vi "PS Control.vi"() -> ()   [LabVIEW 2025]
doc: "Author: Scott Hannahs <sth@magnet.fsu.edu>\n\nThis software is licensed for use under the “MIT License\"\nCopyright (c) 2025 Scott Hannahs, sth@sth@magnet.sthnet.net\n\nPermission is hereby granted, free of charge, to any person obtaining a copy of this software and associated documentation files (the \"Software\"), to deal in the Software without restriction, including without limitation the rights to use, copy, modify, merge, publish, distribute, sublicense, and/or sell copies of the Software, and to permit persons to whom the Software is furnished to do so, subject to the following conditions: The above copyright notice and this permission notice shall be included in all copies or substantial portions of the Software.\n\nTHE SOFTWARE IS PROVIDED \"AS IS\", WITHOUT WARRANTY OF ANY KIND, EXPRESS OR IMPLIED, INCLUDING BUT NOT LIMITED TO THE WARRANTIES OF MERCHANTABILITY, FITNESS FOR A PARTICULAR PURPOSE AND NONINFRINGEMENT. IN NO EVENT SHALL THE AUTHORS OR COPYRIGHT HOLDERS BE LIABLE FOR ANY CLAIM, DAMAGES OR OTHER LIABILITY, WHETHER IN AN ACTION OF CONTRACT, TORT OR OTHERWISE, ARISING FROM, OUT OF OR IN CONNECTION WITH THE SOFTWARE OR THE USE OR OTHER DEALINGS IN THE SOFTWARE."
uses:
  Sub Controls/PS Status.ctl
  PS Comm Globals.vi
panel:
  out "Status":T1
  in  "Slew Rate [T/min]":dbl=1.0 caption="(7.055) Max)" min=0.001 max=50.0 step=0.01 format="%.3f"
  in  "Slew Rate [A/s]":dbl=200.0 caption="(200.0) Max)" min=0.1 max=4000.0 step=10.0 format="%.1f"
  out "Read Loop Ref":refnum<vi>
  out "SC Current [kA]":dbl format="%.5f"
  in  "dup VI reference":refnum<vi>
  in  "Setpoint [kA]":dbl caption="(59.0) Max)" min=-59.0 max=59.0 format="%.5f"
  in  "Setpoint [T]":dbl caption="(34.68) Max)" min=-34.679602421022246 max=34.679602421022246 format="%.5f"
  in  "Pause":bool
  out "Current [kA]":dbl format="%.5f"
  out "Field [T]":dbl caption="Current [kA]" format="%.5f"
  in  "Units":enum32{"tesla", "kAmps"}(radio) caption="tesla            kAmps"
  in  "stop":bool
  in  "Ramp":bool
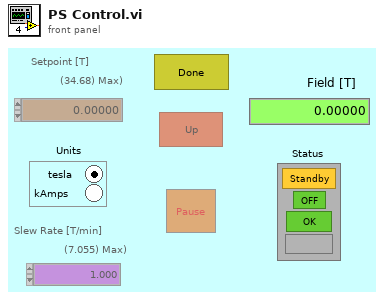
[diagram p1: front panel]
types:
  T1 = typedef "PS Status.ctl" = cluster{"PS On":bool, "PS Fault":bool, "Ramp Status":u16, "Cell Control":bool}
  T2 = cluster{"Control Name":string, "Type Descriptor":i16[], "Flattened Data":string}
  T3 = cluster{"Minimum":dbl, "Maximum":dbl, "Increment":dbl}
  T4 = cluster{string, "type string":i16[], "data string":string}
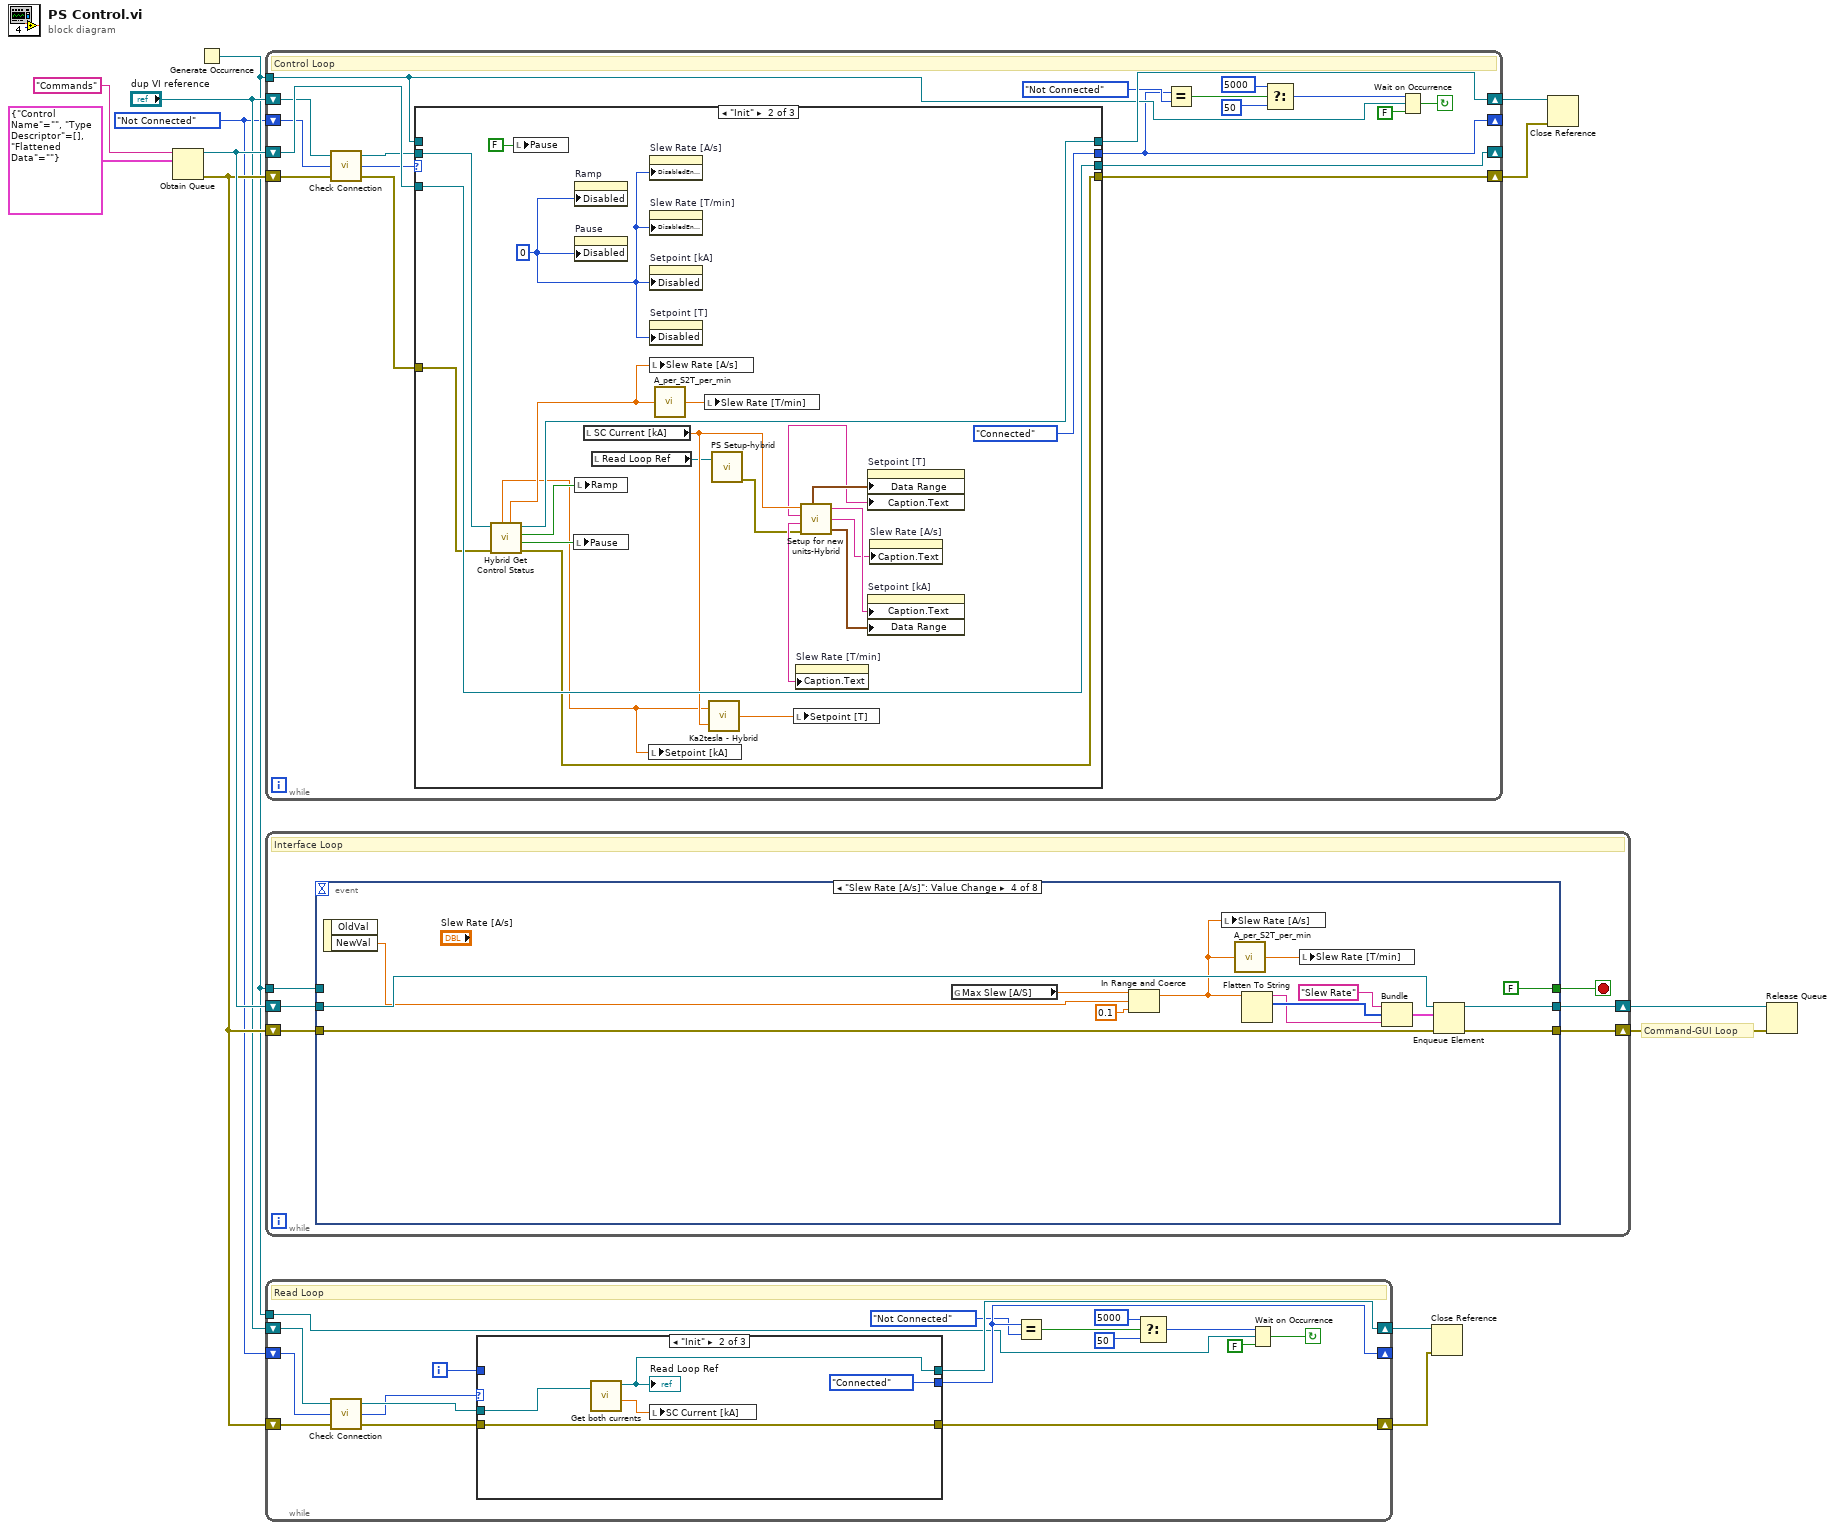
[diagram p0: block diagram]
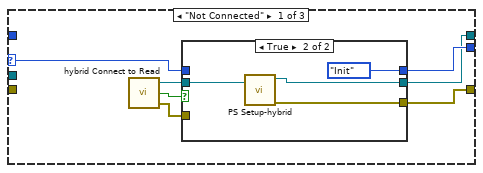
[diagram p2: hidden frame]
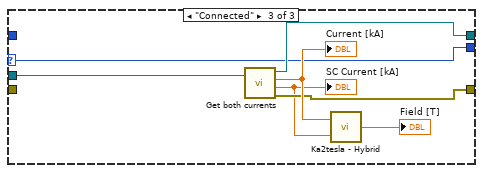
[diagram p4: hidden frame]
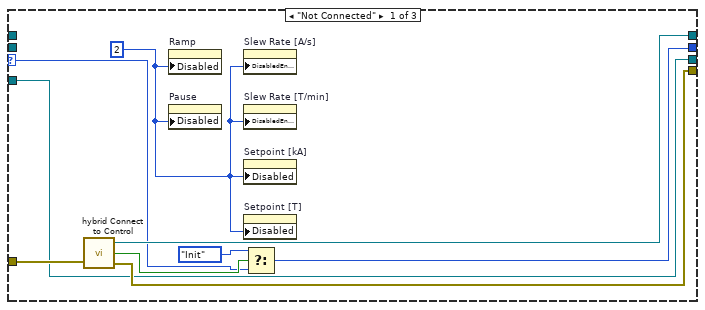
[diagram p5: hidden frame]
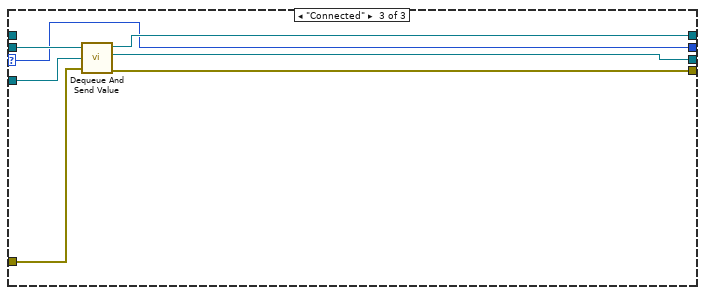
[diagram p6: hidden frame]
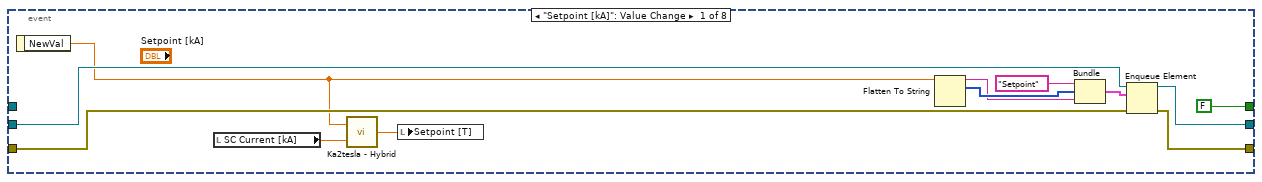
[diagram p7: hidden frame]
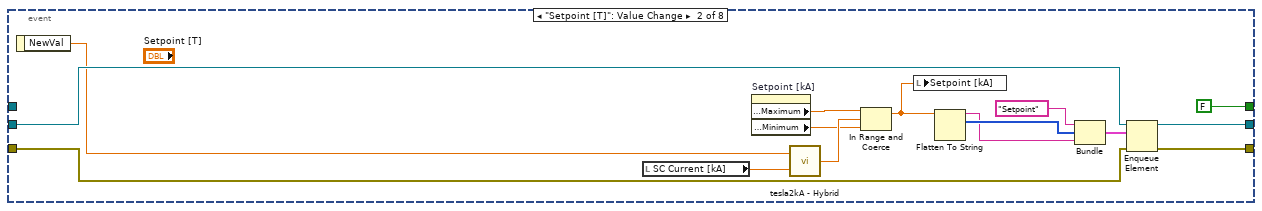
[diagram p8: hidden frame]
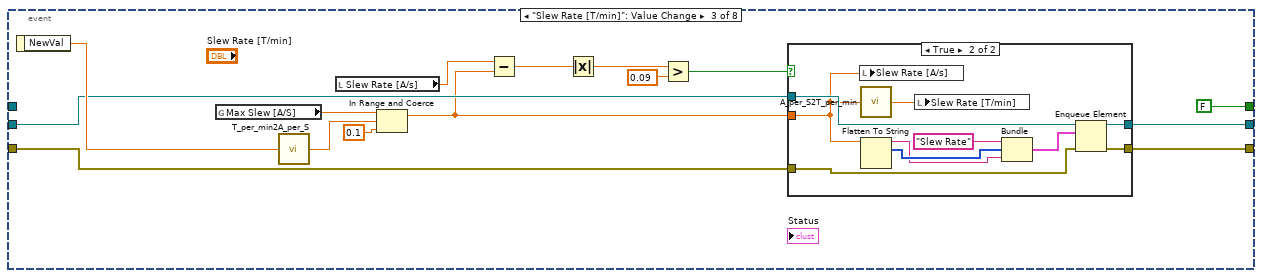
[diagram p9: hidden frame]
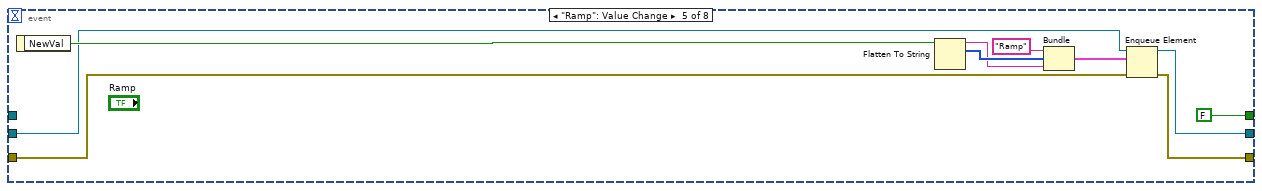
[diagram p11: hidden frame]
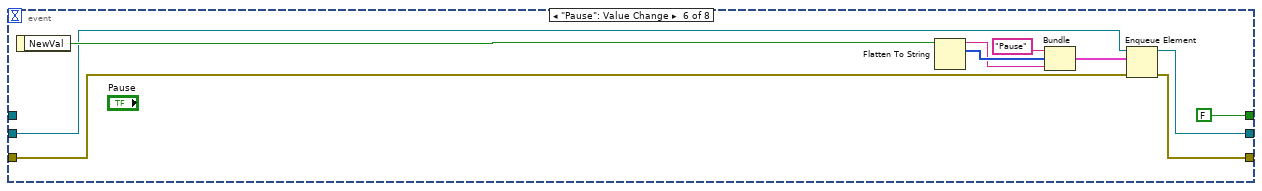
[diagram p12: hidden frame]
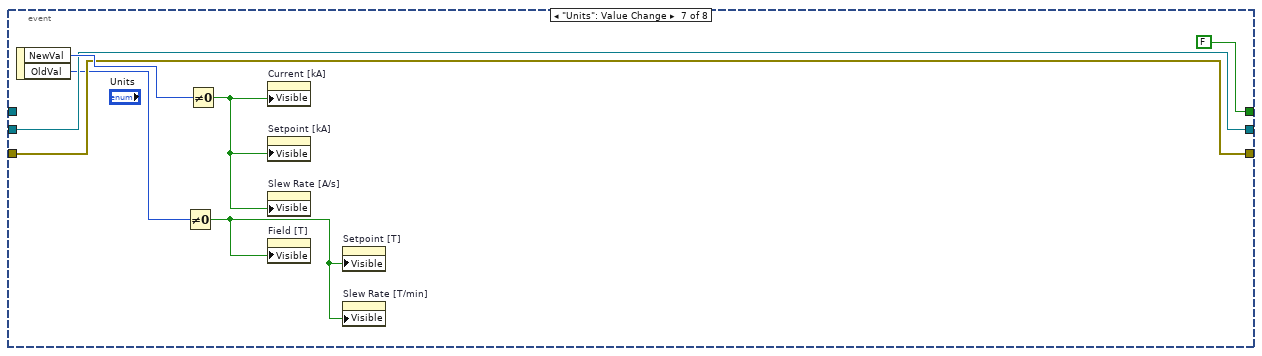
[diagram p13: hidden frame]
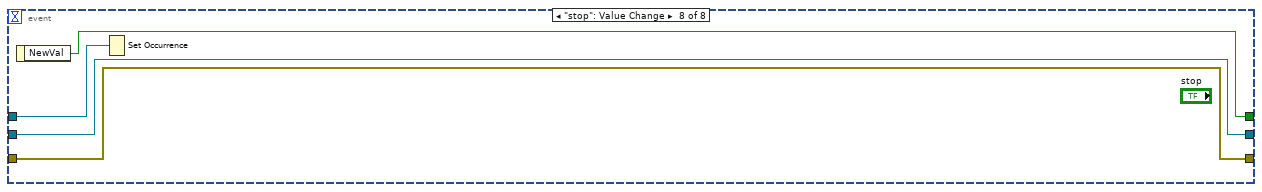
[diagram p14: hidden frame]
diagram:
  w1 = enum16{"Not Connected", "Init", "Connected"}."Not Connected"
  # "Command-GUI Loop"
  n1 = Obtain Queue(name (unnamed)="Commands", element data type=T2 {"Control Name"="", "Type Descriptor"=[], "Flattened Data"=""}) -> (queue out=w11:refnum<queue>, error out=w6:errorcluster)  [unwired: 3 in, 1 out]
  n2 = Generate Occurrence() -> (w2:refnum<k4>)
  n3 = while {
    shift-right: [w32] -> w8
    shift-left: "dup VI reference" -> [w27]
    shift-right: [w31] -> w7
    shift-left: w6 -> [w26]
    shift-right: [w29] -> _
    shift-left: w11 -> [w30]
    tunnel: w2 -> [w22]
    shift-right: [w15] -> _
    shift-left: w1 -> [w24]
    stop <- w21 continue-if-true
    # "Control Loop"
    n4 = call "Check Connection.vi"("error In"=w26, "State In"=w24, "VI reference"=w27) -> ("error out"=w25:errorcluster, "State Out"=w23:enum16{"Not Connected", "Init", "Connected"}, "dup VI reference"=w28:refnum<vi>)
    n5 = case shown="\"Init\"" w23 {
      selector: w23 -> [w35 _ w65]
      tunnel: [w41 w54 w66] -> w32
      tunnel: w25 -> [w40 w53 w69]
      tunnel: [w39 w52 w67] -> w31
      tunnel: w30 -> [w38 w63 w71]
      tunnel: [w38 w63 w70] -> w29
      tunnel: w28 -> [_ w64 w68]
      tunnel: w22 -> [_ _ _]
      tunnel: [w34 enum16{"Not Connected", "Init", "Connected"}."Connected" ("f") w65] -> w15
      frame "Not Connected" {
        w33 = u8 2 ("Disabled")
        n6 = call "hybrid Connect to Control.vi"("error in"=w40) -> ("VI Refnum"=w41:refnum<vi>, "Success"=w37:bool, "error out"=w39:errorcluster)  [unwired: 1 in]
        n7 = property on="Ramp" class="Bool (strict)"("Disabled"=w33) -> ()  [unwired: 2 in, 2 out]
        n8 = property on="Pause" class="Bool (strict)"("Disabled"=w33) -> ()  [unwired: 2 in, 2 out]
        n9 = property on="Slew Rate [A/s]" class="DigNum (strict)"("DisabledEnum"=w33) -> ()  [unwired: 2 in, 2 out]
        n10 = property on="Slew Rate [T/min]" class="DigNum (strict)"("DisabledEnum"=w33) -> ()  [unwired: 2 in, 2 out]
        n11 = property on="Setpoint [kA]" class="DigNum (strict)"("Disabled"=w33) -> ()  [unwired: 2 in, 2 out]
        n12 = property on="Setpoint [T]" class="DigNum (strict)"("Disabled"=w33) -> ()  [unwired: 2 in, 2 out]
        n13 = Select(t=enum16{"Not Connected", "Init", "Connected"}."Init", s=w37, f=w35) -> (s? t:f=w34:enum16{"Not Connected", "Init", "Connected"})
      }
      frame "Init" {
        w49 = u8 0 ("Disabled")
        n14 = call "Hybrid Get Control Status.vi"("error in (no error)"=w53, "VI in"=w64) -> ("error out"=w52:errorcluster, "Pause"=w50:bool, "Ramp"=w51:bool, "VI out"=w54:refnum<vi>, "Slew Rate [A/s]"=w45:dbl, "Setpoint"=w44:dbl)  [unwired: 4 in]
        n15 = local write "Pause"(FALSE ("Pause")) -> ()
        n16 = local write "Pause"(w50) -> ()
        n17 = property on="Ramp" class="Bool (strict)"("Disabled"=w49) -> ()  [unwired: 2 in, 2 out]
        n18 = property on="Pause" class="Bool (strict)"("Disabled"=w49) -> ()  [unwired: 2 in, 2 out]
        n19 = local write "Ramp"(w51) -> ()
        n20 = local read "SC Current [kA]"() -> (w61:dbl)
        n21 = local read "Read Loop Ref"() -> (w43:refnum<vi>)
        n22 = local write "Setpoint [kA]"(w44) -> ()
        n23 = property on="Slew Rate [A/s]" class="DigNum (strict)"("DisabledEnum"=w49) -> ()  [unwired: 2 in, 2 out]
        n24 = property on="Slew Rate [T/min]" class="DigNum (strict)"("DisabledEnum"=w49) -> ()  [unwired: 2 in, 2 out]
        n25 = property on="Setpoint [kA]" class="DigNum (strict)"("Disabled"=w49) -> ()  [unwired: 2 in, 2 out]
        n26 = property on="Setpoint [T]" class="DigNum (strict)"("Disabled"=w49) -> ()  [unwired: 2 in, 2 out]
        n27 = local write "Slew Rate [A/s]"(w45) -> ()
        n28 = call "A_per_S2T_per_min.vi"("A/sec"=w45) -> ("T/min"=w46:dbl)
        n29 = local write "Slew Rate [T/min]"(w46) -> ()
        n30 = call "Ka2tesla - Hybrid.vi"("SC Current [kA]"=w61, "Current [KA]"=w44) -> ("Field"=w56:dbl)
        n31 = call "PS Setup-hybrid.vi"("vi reference"=w43) -> ("error out"=w42:errorcluster)  [unwired: 4 in, 2 out]
        n32 = local write "Setpoint [T]"(w56) -> ()
        n33 = call "Setup for new units-Hybrid.vi"("SC Current [kA]"=w61, "error in (no error)"=w42) -> ("Field Setpoint Caption"=w57:string, "Field Slew Rate Caption"=w47:string, "Field Range"=w58:T3, "Current Setpoint Caption"=w60:string, "Current Slew Rate Caption"=w48:string, "Current Range"=w59:T3)
        n34 = property on="Slew Rate [T/min]" class="DigNum (strict)"("Caption.Text"=w47) -> ()  [unwired: 2 in, 2 out]
        n35 = property on="Setpoint [T]" class="DigNum (strict)"("Data Range"=w58, "Caption.Text"=w57) -> ()  [unwired: 2 in, 2 out]
        n36 = property on="Setpoint [kA]" class="DigNum (strict)"("Caption.Text"=w60, "Data Range"=w59) -> ()  [unwired: 2 in, 2 out]
        n37 = property on="Slew Rate [A/s]" class="DigNum (strict)"("Caption.Text"=w48) -> ()  [unwired: 2 in, 2 out]
      }
      frame "Connected" {
        n38 = call "Dequeue And Send Value.vi"("VI reference"=w68, "queue in"=w71, "error in"=w69) -> ("dup VI Refnum"=w66:refnum<vi>, "queue out"=w70:refnum<queue>, "error out"=w67:errorcluster)  [unwired: 1 out]
      }
    }
    n39 = Equal?(x=w15, y=enum16{"Not Connected", "Init", "Connected"}."Not Connected") -> (x = y?=w16:bool)
    n40 = Select(t=5000 ("ms timeout (-1)"), s=w16, f=50 ("ms timeout (-1)")) -> (s? t:f=w14:i32)
    n41 = Wait on Occurrence(1:FALSE ("ignore previous (T)"), 2:w22, 3:w14) -> (0:w21:bool)
  }
  n42 = while {
    tunnel: w2 -> [w76]
    shift-right: [w74] -> w9
    shift-left: w11 -> [w75]
    shift-right: [w72] -> w10
    shift-left: w6 -> [w73]
    stop <- w77 stop-if-true
    # "Interface Loop"
    n43 = event shown="[3] \"Slew Rate [A/s]\": Value Change" {
      selector: _ -> [_ _ _ _ _ _ _ _]
      dyn-events: _ -> [_ _ _ _ _ _ _ _]
      timeout: _ -> [_ _ _ _ _ _ _ _]
      tunnel: [FALSE ("NewVal") FALSE ("NewVal") FALSE ("NewVal") FALSE ("NewVal") FALSE ("NewVal") FALSE ("NewVal") FALSE ("NewVal") w176] -> w77
      tunnel: w73 -> [w84 w99 w115 w140 w150 w160 w170 w173]
      tunnel: w76 -> [_ _ _ _ _ _ _ w175]
      tunnel: w75 -> [w87 w102 w113 w144 w152 w162 w171 w174]
      tunnel: [w85 w100 w112 w141 w151 w161 w171 w174] -> w74
      tunnel: [w83 w98 w114 w139 w149 w159 w170 w173] -> w72
      event "Setpoint [kA]": Value Change {
        n44 = event-data() -> ("NewVal"=w79:dbl)  [unwired: 1 in]
        n45 = local read "SC Current [kA]"() -> (w78:dbl)
        n46 = call "Ka2tesla - Hybrid.vi"("SC Current [kA]"=w78, "Current [KA]"=w79) -> ("Field"=w80:dbl)
        n47 = local write "Setpoint [T]"(w80) -> ()
        n48 = Flatten To String(anything=w79) -> (data string=w88:string, type string=w89:i16[])  [unwired: 3 in, 1 out]
        n49 = Bundle("Setpoint", "type string"=w89, "data string"=w88) -> (w86:T4)  [unwired: 1 in]
        n50 = Enqueue Element(queue=w87, element=w86, error in (no error)=w84) -> (queue out=w85:refnum<queue>, error out=w83:errorcluster)  [unwired: 1 in, 1 out]
      }
      event "Setpoint [T]": Value Change {
        n51 = event-data() -> ("NewVal"=w95:dbl)  [unwired: 1 in]
        n52 = local read "SC Current [kA]"() -> (w90:dbl)
        n53 = property on="Setpoint [kA]" class="DigNum (strict)"() -> ("Data Range:Maximum"=w92:dbl, "Data Range:Minimum"=w91:dbl)  [unwired: 2 in, 2 out]
        n54 = call "tesla2kA - Hybrid.vi"("SC Current [kA]"=w90, "Magnet Field [T]"=w95) -> ("Current [kA]"=w94:dbl)
        n55 = In Range and Coerce(upper limit=w92, x=w94, lower limit=w91) -> (coerced(x)=w93:dbl)  [unwired: 1 out]
        n56 = local write "Setpoint [kA]"(w93) -> ()
        n57 = Flatten To String(anything=w93) -> (data string=w103:string, type string=w104:i16[])  [unwired: 3 in, 1 out]
        n58 = Bundle("Setpoint", "type string"=w104, "data string"=w103) -> (w101:T4)  [unwired: 1 in]
        n59 = Enqueue Element(queue=w102, element=w101, error in (no error)=w99) -> (queue out=w100:refnum<queue>, error out=w98:errorcluster)  [unwired: 1 in, 1 out]
      }
      event "Slew Rate [T/min]": Value Change {
        n60 = event-data() -> ("NewVal"=w119:dbl)  [unwired: 1 in]
        n61 = global read "PS Comm Globals.vi" "Max Slew [A/S]"() -> (w117:dbl)
        n62 = call "T_per_min2A_per_S.vi"("T/min"=w119) -> ("A/sec"=w116:dbl)
        n63 = local read "Slew Rate [A/s]"() -> (w109:dbl)
        n64 = In Range and Coerce(upper limit=w117, x=w116, lower limit=0.1) -> (coerced(x)=w110:dbl)  [unwired: 1 out]
        n65 = Subtract(x=w109, y=w110) -> (x-y=w108:dbl)
        n66 = Absolute Value(x=w108) -> (abs(x)=w107:dbl)
        n67 = Greater?(x=w107, y=0.09) -> (0:w105:bool)
        n68 = case shown="True" w105 {
          tunnel: w115 -> [w120 w126]
          tunnel: [w120 w125] -> w114
          tunnel: w113 -> [w121 w124]
          tunnel: [w121 w123] -> w112
          tunnel: w110 -> [_ w122]
          frame False {
          }
          frame True {
            n69 = local write "Slew Rate [A/s]"(w122) -> ()
            n70 = call "A_per_S2T_per_min.vi"("A/sec"=w122) -> ("T/min"=w131:dbl)
            n71 = Flatten To String(anything=w122) -> (data string=w129:string, type string=w130:i16[])  [unwired: 3 in, 1 out]
            n72 = local write "Slew Rate [T/min]"(w131) -> ()
            n73 = Bundle("Slew Rate", "type string"=w130, "data string"=w129) -> (w127:T4)  [unwired: 1 in]
            n74 = Enqueue Element(queue=w124, element=w127, error in (no error)=w126) -> (queue out=w123:refnum<queue>, error out=w125:errorcluster)  [unwired: 1 in, 1 out]
          }
        }
      }
      event "Slew Rate [A/s]": Value Change {
        n75 = event-data() -> ("NewVal"=w143:dbl)  [unwired: 1 in, 1 out]
        n76 = global read "PS Comm Globals.vi" "Max Slew [A/S]"() -> (w133:dbl)
        n77 = In Range and Coerce(upper limit=w133, x=w143, lower limit=0.1) -> (coerced(x)=w134:dbl)  [unwired: 1 out]
        n78 = local write "Slew Rate [A/s]"(w134) -> ()
        n79 = call "A_per_S2T_per_min.vi"("A/sec"=w134) -> ("T/min"=w145:dbl)
        n80 = Flatten To String(anything=w134) -> (data string=w137:string, type string=w138:i16[])  [unwired: 3 in, 1 out]
        n81 = local write "Slew Rate [T/min]"(w145) -> ()
        n82 = Bundle("Slew Rate", "type string"=w138, "data string"=w137) -> (w135:T4)  [unwired: 1 in]
        n83 = Enqueue Element(queue=w144, element=w135, error in (no error)=w140) -> (queue out=w141:refnum<queue>, error out=w139:errorcluster)  [unwired: 1 in, 1 out]
      }
      event "Ramp": Value Change {
        n84 = event-data() -> ("NewVal"=w155:bool)  [unwired: 1 in]
        n85 = Flatten To String(anything=w155) -> (data string=w153:string, type string=w154:i16[])  [unwired: 3 in, 1 out]
        n86 = Bundle("Ramp", "type string"=w154, "data string"=w153) -> (w147:T4)  [unwired: 1 in]
        n87 = Enqueue Element(queue=w152, element=w147, error in (no error)=w150) -> (queue out=w151:refnum<queue>, error out=w149:errorcluster)  [unwired: 1 in, 1 out]
      }
      event "Pause": Value Change {
        n88 = event-data() -> ("NewVal"=w165:bool)  [unwired: 1 in]
        n89 = Flatten To String(anything=w165) -> (data string=w163:string, type string=w164:i16[])  [unwired: 3 in, 1 out]
        n90 = Bundle("Pause", "type string"=w164, "data string"=w163) -> (w157:T4)  [unwired: 1 in]
        n91 = Enqueue Element(queue=w162, element=w157, error in (no error)=w160) -> (queue out=w161:refnum<queue>, error out=w159:errorcluster)  [unwired: 1 in, 1 out]
      }
      event "Units": Value Change {
        n92 = event-data() -> ("NewVal"=w172:enum32{"tesla", "kAmps"}, "OldVal"=w168:enum32{"tesla", "kAmps"})  [unwired: 1 in]
        n93 = Not Equal To 0?(x=w168) -> (x != 0?=w167:bool)
        n94 = Not Equal To 0?(x=w172) -> (x != 0?=w166:bool)
        n95 = property on="Current [kA]" class="DigNum (strict)"("Visible"=w166) -> ()  [unwired: 2 in, 2 out]
        n96 = property on="Setpoint [kA]" class="DigNum (strict)"("Visible"=w166) -> ()  [unwired: 2 in, 2 out]
        n97 = property on="Slew Rate [A/s]" class="DigNum (strict)"("Visible"=w166) -> ()  [unwired: 2 in, 2 out]
        n98 = property on="Field [T]" class="DigNum (strict)"("Visible"=w167) -> ()  [unwired: 2 in, 2 out]
        n99 = property on="Setpoint [T]" class="DigNum (strict)"("Visible"=w167) -> ()  [unwired: 2 in, 2 out]
        n100 = property on="Slew Rate [T/min]" class="DigNum (strict)"("Visible"=w167) -> ()  [unwired: 2 in, 2 out]
      }
      event "stop": Value Change {
        n101 = event-data() -> ("NewVal"=w176:bool)  [unwired: 1 in]
        n102 = Set Occurrence(w175) -> ()
      }
    }
  }
  n103 = while {
    shift-right: [w184] -> _
    shift-left: w1 -> [w188]
    shift-right: [w193] -> w3
    shift-left: "dup VI reference" -> [w191]
    shift-right: [w194] -> w4
    shift-left: w6 -> [w189]
    tunnel: w2 -> [w180]
    i -> [w177]
    stop <- w179 continue-if-true
    # "Read Loop"
    n104 = call "Check Connection.vi"("error In"=w189, "State In"=w188, "VI reference"=w191) -> ("error out"=w190:errorcluster, "State Out"=w187:enum16{"Not Connected", "Init", "Connected"}, "dup VI reference"=w192:refnum<vi>)
    n105 = case shown="\"Init\"" w187 {
      selector: w187 -> [w198 _ w215]
      tunnel: [w195 w209 w217] -> w193
      tunnel: [w199 w213 w216] -> w194
      tunnel: [w197 enum16{"Not Connected", "Init", "Connected"}."Connected" ("f") w215] -> w184
      tunnel: w192 -> [_ w210 w218]
      tunnel: w190 -> [_ w213 _]
      tunnel: w177 -> [_ _ _]
      frame "Not Connected" {
        n106 = call "hybrid Connect to Read.vi"() -> ("VI Refnum"=w196:refnum<vi>, "Success"=w201:bool, "error out"=w200:errorcluster)  [unwired: 2 in]
        n107 = case shown="True" w201 {
          tunnel: w200 -> [w204 _]
          tunnel: [w204 w206] -> w199
          tunnel: w198 -> [w203 _]
          tunnel: [w203 enum16{"Not Connected", "Init", "Connected"}."Init"] -> w197
          tunnel: w196 -> [w202 w205]
          tunnel: [w202 w207] -> w195
          frame False {
          }
          frame True {
            n108 = call "PS Setup-hybrid.vi"("vi reference"=w205) -> ("dup VI reference"=w207:refnum<vi>, "error out"=w206:errorcluster)  [unwired: 4 in, 1 out]
          }
        }
      }
      frame "Init" {
        n109 = call "Get both currents.vi"("VI reference"=w210) -> ("SC Current [kA]"=w211:dbl, "dup VI reference"=w209:refnum<vi>)  [unwired: 1 in, 3 out]
        "Read Loop Ref" <- w209
        n110 = local write "SC Current [kA]"(w211) -> ()
      }
      frame "Connected" {
        n111 = call "Get both currents.vi"("VI reference"=w218) -> ("error out"=w216:errorcluster, "SC Current [kA]"=w214:dbl, "Current [KA]"=w219:dbl, "dup VI reference"=w217:refnum<vi>)  [unwired: 1 in, 1 out]
        "Current [kA]" <- w219
        "SC Current [kA]" <- w214
        n112 = call "Ka2tesla - Hybrid.vi"("SC Current [kA]"=w214, "Current [KA]"=w219) -> ("Field"=→"Field [T]":dbl)
      }
    }
    n113 = Equal?(x=w184, y=enum16{"Not Connected", "Init", "Connected"}."Not Connected") -> (x = y?=w186:bool)
    n114 = Select(t=5000 ("ms timeout (-1)"), s=w186, f=50 ("ms timeout (-1)")) -> (s? t:f=w185:i32)
    n115 = Wait on Occurrence(1:FALSE ("ignore previous (T)"), 2:w180, 3:w185) -> (0:w179:bool)
  }
  n116 = Close Reference(reference=w3, error in (no error)=w4) -> ()  [unwired: 1 out]
  n117 = Close Reference(reference=w8, error in (no error)=w7) -> ()  [unwired: 1 out]
  n118 = Release Queue(queue=w9, error in (no error)=w10) -> ()  [unwired: 1 in, 3 out]
